vi "runTestScenario.vi"(8 "error in (no error)":errorcluster, 11 "ITestScenario in":refnum<class "ITestScenario.lvclass">) -> (0 "error out":errorcluster, 2 "TestExecution":T1, 3 "ITestScenario out":refnum<class "ITestScenario.lvclass">)   [LabVIEW 2015, in "ITestScenario.lvclass"]
uses:
  ITestScenario.lvclass
  Typedefs/TestExecution.ctl
  Typedefs/ILCBTTypedefs.lvlib
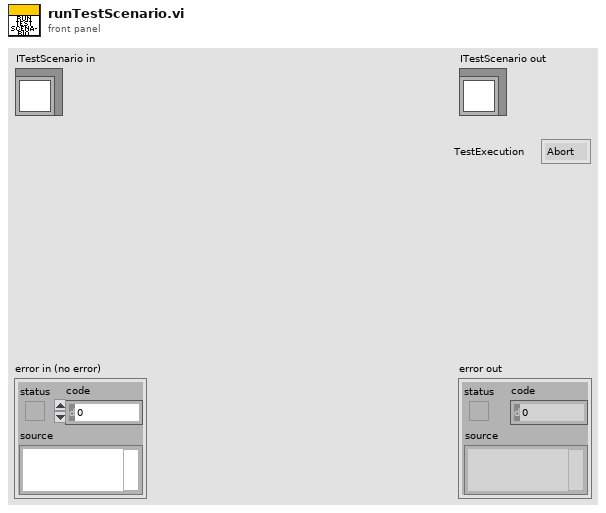
[diagram p1: front panel]
types:
  T1 = typedef "ILCBTTypedefs.lvlib/TestExecution.ctl" = enum16{"Abort", "Continue"}
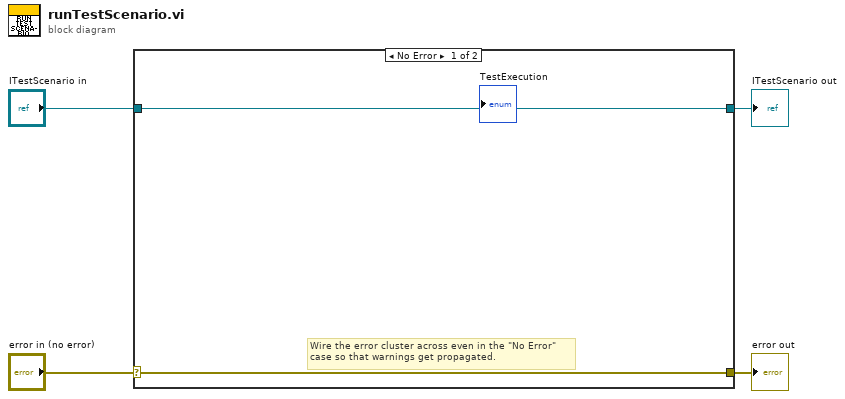
[diagram p0: block diagram]
diagram:
  n1 = case shown="No Error" "error in (no error)" {
    selector: "error in (no error)" -> [w5 w8]
    tunnel: [w5 w8] -> w3
    tunnel: [w6 w7] -> w1
    tunnel: "ITestScenario in" -> [w6 w7]
    frame No Error {
      # "Wire the error cluster across even in the \"No Error\"\ncase so that warnings get propagated."
    }
    frame Error {
    }
  }
  "error out" <- w3
  "ITestScenario out" <- w1
